vi "SeCrTs-DO waveform Samples bulider .vi"(7 "Samples 2":i32=10, 9 "Data input 2":waveform(dbl)[](array[waveform]), 11 "DO_Data RD":refnum<queue>) -> (1 "Array 4":timestamp[][](array[timestamp]), 2 "Array 3":dbl[][](array[numeric]), 4 "Wave out":waveform(dbl)[][](array[waveform]))   [LabVIEW 2022 SP3]
panel:
  out "Array 5":waveform(dbl)[](array[waveform])
  out "overflow?":bool
  out "Array 2":waveform(dbl)[](array[waveform])
  out "Array":waveform(dbl)[][](array[waveform])
  out "transposed array":waveform(dbl)[][](array[waveform])
  out "Data out 3":waveform(dbl)[](array[waveform])
  in  "Data input 3":waveform(dbl)[](array[waveform])
  out "Data out 2":waveform(dbl)[](array[waveform])
  out "overflow? 2":bool
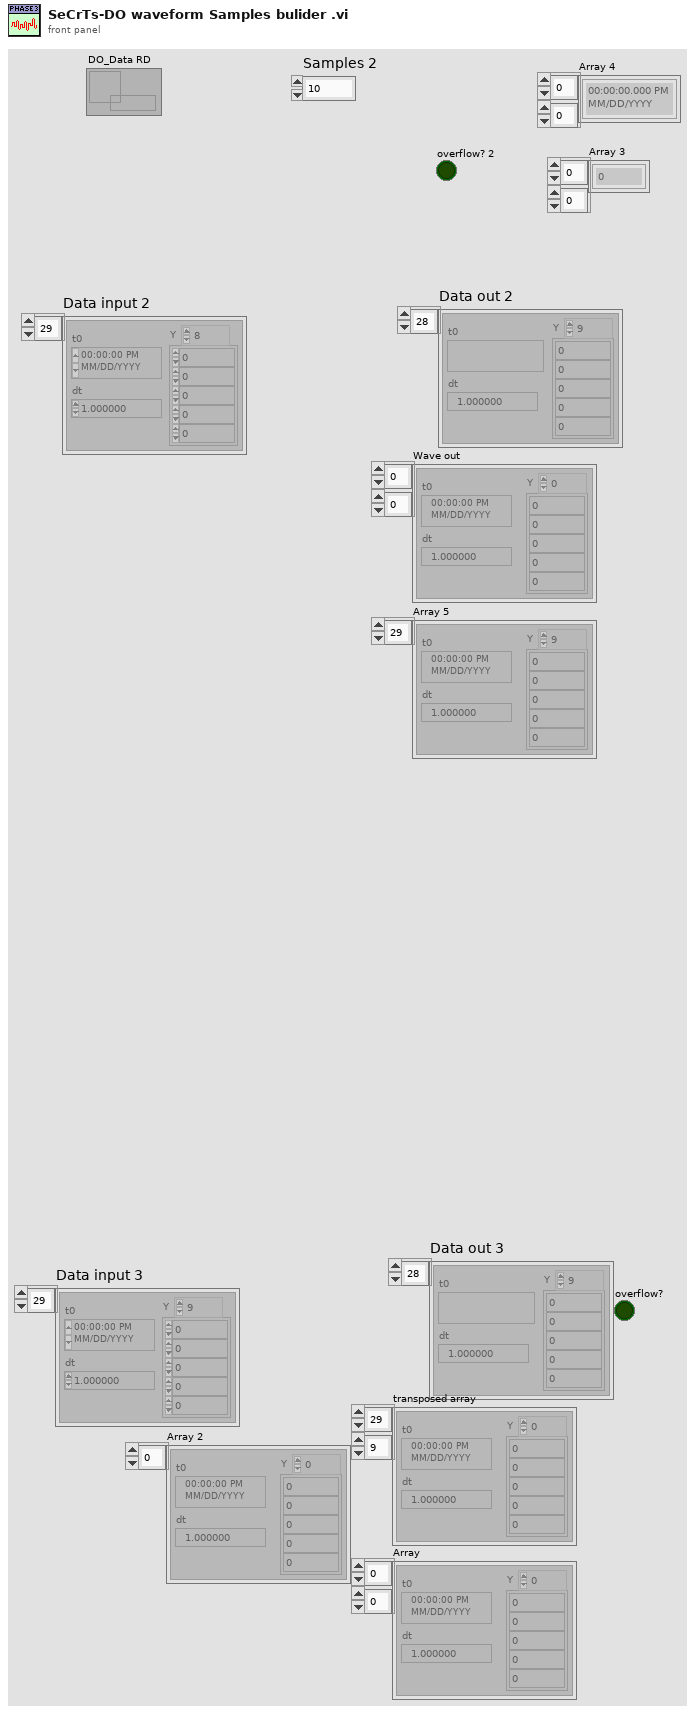
[diagram p1: front panel]
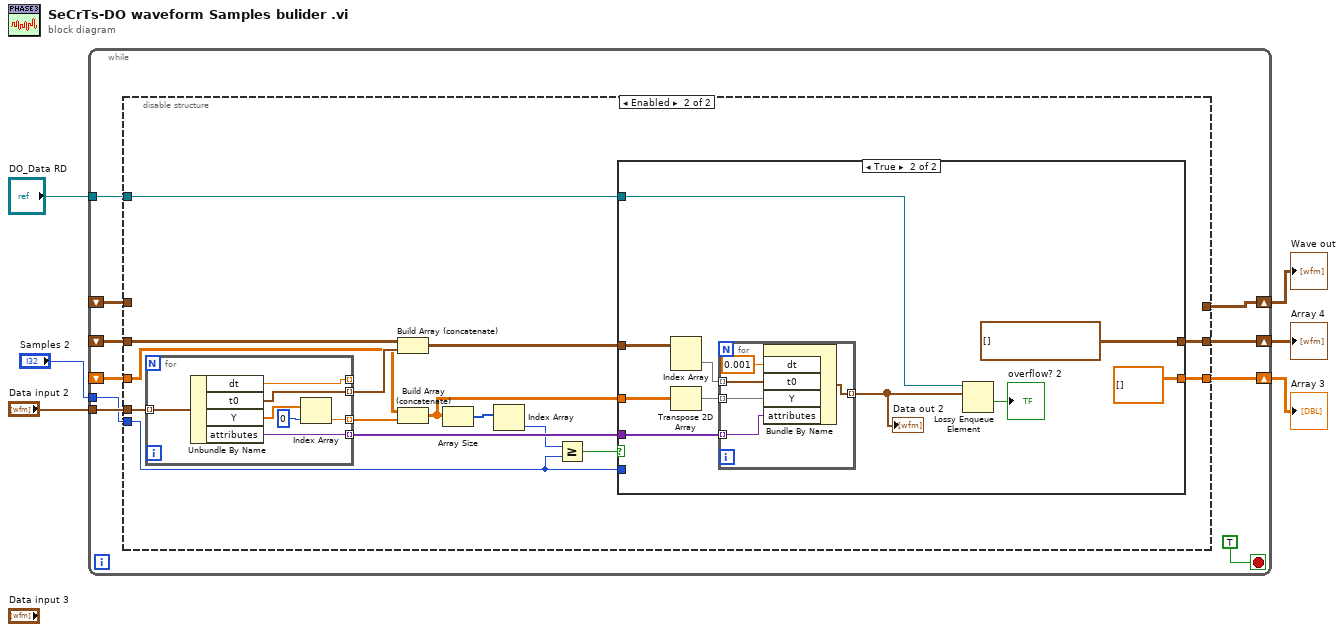
[diagram p0: block diagram]
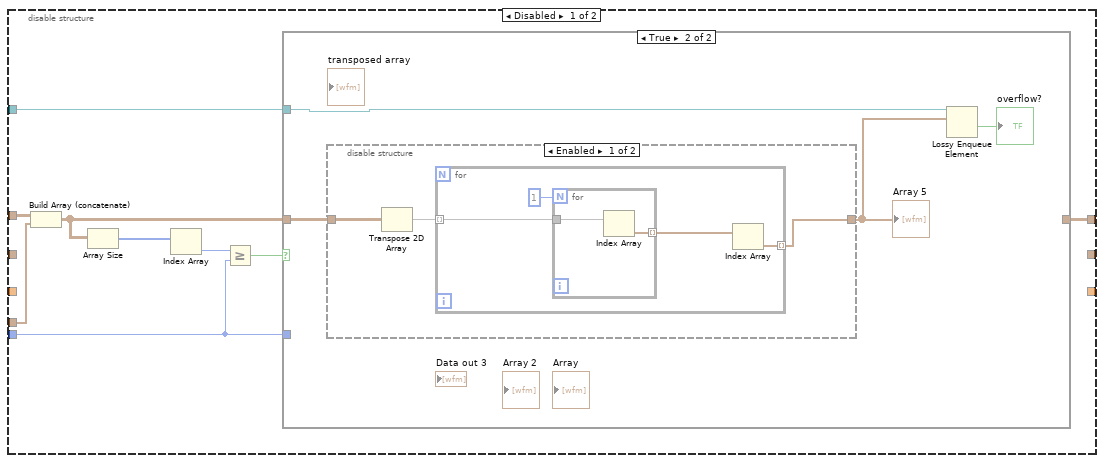
[diagram p2: hidden frame]
diagram:
  n1 = while {
    tunnel: "Data input 2" -> [w12]
    tunnel: "Samples 2" -> [w11]
    tunnel: "DO_Data RD" -> [w8]
    shift-right: [w13] -> w5
    shift-left: _ -> [w16]
    shift-right: [w14] -> w6
    shift-left: _ -> [w15]
    shift-right: [w9] -> w2
    shift-left: _ -> [w10]
    stop <- TRUE stop-if-true
    n2 = disable-structure shown="Enabled" {
      disable-tunnel: w8 -> [w18 w55]
      disable-tunnel: w16 -> [_ w46]
      disable-tunnel: w15 -> [_ w45]
      disable-tunnel: [_ w44] -> w14
      disable-tunnel: [_ w43] -> w13
      disable-tunnel: w12 -> [w22 w42]
      disable-tunnel: w11 -> [w23 w41]
      disable-tunnel: w10 -> [w21 _]
      disable-tunnel: [w17 _] -> w9
      frame Disabled {
        n3 = Build Array (concatenate)(w21, w22) -> (w25:waveform(dbl)[][])
        n4 = Array Size(array=w25) -> (size(s)=w20:i32[])
        n5 = Index Array(array=w20) -> (element=w19:i32)  [unwired: 1 in]
        n6 = Greater Or Equal?(x=w19, y=w23) -> (x >= y?=w24:bool)
        n7 = case shown="True" w24 {
          tunnel: w25 -> [w26 w29]
          tunnel: [w26 _] -> w17
          tunnel: w23 -> [_ _]
          tunnel: w18 -> [_ w28]
          frame False {
          }
          frame True {
            n8 = disable-structure shown="Enabled" {
              disable-tunnel: w29 -> [w32 w40]
              disable-tunnel: [w31 w40] -> w27
              frame Enabled {
                n9 = Transpose 2D Array(2D array=w32) -> (transposed array=w33:waveform(dbl)[][])
                n10 = for {
                  tunnel: [w35] -> w31 mode=indexing
                  tunnel: w33 -> [w34] mode=indexing
                  n11 = for {
                    N: 1 -> [_]
                    tunnel: w34 -> [w39]
                    tunnel: [w38] -> w36 mode=indexing
                    n12 = Index Array(array=w39) -> (element=w38:waveform(dbl))  [unwired: 1 in]
                  }
                  n13 = Index Array(array=w36) -> (element=w35:waveform(dbl))  [unwired: 1 in]
                }
              }
              frame Disabled {
              }
            }
            "Array 5" <- w27
            n14 = Lossy Enqueue Element(queue=w28, element=w27) -> (overflow?=→"overflow?":bool)  [unwired: 1 in, 3 out]
          }
        }
      }
      frame Enabled {
        n15 = for {
          tunnel: w42 -> [w79] mode=indexing
          tunnel: [w77] -> w47 mode=indexing
          tunnel: [w75] -> w52 mode=indexing
          tunnel: [w74] -> w54 mode=indexing
          tunnel: [w73] -> _ mode=indexing
          n16 = Unbundle By Name(w79) -> ("dt"=w73:dbl, "t0"=w75:timestamp, "Y"=w78:dbl[], "attributes"=w74:variant)
          n17 = Index Array(array=w78, index=0) -> (element=w77:dbl)
        }
        n18 = Build Array (concatenate)(w45, w52) -> (w53:timestamp[][])
        n19 = Build Array (concatenate)(w46, w47) -> (w50:dbl[][])
        n20 = Array Size(array=w50) -> (size(s)=w48:i32[])
        n21 = Index Array(array=w48) -> (element=w49:i32)  [unwired: 1 in]
        n22 = Greater Or Equal?(x=w49, y=w41) -> (x >= y?=w51:bool)
        n23 = case shown="True" w51 {
          tunnel: w50 -> [w57 w62]
          tunnel: [w57 dbl[][] []] -> w43
          tunnel: w53 -> [w56 w59]
          tunnel: [w56 timestamp[][] []] -> w44
          tunnel: w54 -> [_ w67]
          tunnel: w41 -> [_ _]
          tunnel: w55 -> [_ w65]
          frame False {
          }
          frame True {
            n24 = Index Array(array=w59) -> (element=w58:timestamp[])  [unwired: 2 in]
            n25 = Transpose 2D Array(2D array=w62) -> (transposed array=w66:dbl[][])
            n26 = for {
              tunnel: w66 -> [w72] mode=indexing
              tunnel: w67 -> [w71] mode=indexing
              tunnel: [w70] -> w64 mode=indexing
              tunnel: w58 -> [w69] mode=indexing
              n27 = Bundle By Name("dt"=0.001, "t0"=w69, "Y"=w72, "attributes"=w71) -> (w70:waveform(dbl))  [unwired: 1 in]
            }
            "Data out 2" <- w64
            n28 = Lossy Enqueue Element(queue=w65, element=w64) -> (overflow?=→"overflow? 2":bool)  [unwired: 1 in, 3 out]
          }
        }
      }
    }
  }
  "Array 4" <- w6
  "Array 3" <- w5
  "Wave out" <- w2
